vi "Open_File_for_write.vi"(8 "advisory dialog? (display:T)":bool=TRUE, 9 "append to file? (new file:F)":bool, 11 "file path":path) -> (0 "error out":errorcluster, 3 "refnum":refnum<file>)   [LabVIEW 2010]
doc: "Opens an existing file, creates a new file, or replaces an existing file, programmatically or interactively using dialog. You can optionally specify a dialog prompt, default file name, start path, or filter pattern, and you can specify open and deny modes when opening a file, plus group and permission when creating a new file. Use this VI with the intermediate Write File+ or Read File+ VIs described below.\n\nfile path is the path name of the file. If file path is empty (default value) or is Not A Path, the VI displays a File dialog box from which you can select a file. Error 43 occurs if the user cancels the dialog. \n\nfunction is the operation to perform:\n\n 0 (open) opens an existing file. Error 7 occurs if the file cannot be found.\n \n 1 (open or create) opens an existing file or creates a new file if one does not exist.\n\n 2 (create or replace) creates a new file or replaces a file if it exists and you give permission. Replacement is done by opening the file and setting EOF to 0. Error 43 occurs if the user elects to disallow the replacement using dialog. \n\n 3 (create) creates a new file. Error 8 occurs if the file already exists.\n\nadvisory dialog? Set TRUE (default) if you want a dialog if function=0 and the file does not exist, or if function=2 or 3 and the file exists.\n\nprompt is the message that appears below the list of files and directories in the file dialog.\n\ndefault name is the initial file name that appears in the selection box of the file dialog.\n\nstart path is the path name to the initially displayed directory in a file dialog. The default value is Not A Path, which is the path to the last directory shown in a file dialog.\n\npattern is the match pattern specification to display only certain types of files or directories. See the description of the File Dialog function for more information.\n\nerror in is a cluster of three elements (error?, code, and source) that describe the upstream error state, that is, the existance of any error preceeding the execution of the VI. The VI executes normally only if no incoming error exists; otherwise it merely passes the error in value to error out. error? is TRUE if an error occurred; the default value is FALSE. code is the error code; the default value is 0. source is in most cases the name of the VI or function that produced the error; the default value is an empty string.\n\nnew file path is the path of the file opened or created. You can use this output to determine the path of a file that you open or create using dialog. new file path returns Not A Path if the user selects Cancel from the dialog box.\n\nrefnum is the reference number of the open file. The value is Not A Refnum if the file cannot be opened.\n\nfile size is the size of the file in bytes; it is also the location of the end of file.\n\nerror out is a cluster of three elements (error?, code, and source) that describe the error state following the execution of the VI. If an incoming error does not exist, the VI executes normally and error out describes the VI's error state; if an incoming error exists, error out equals error in."
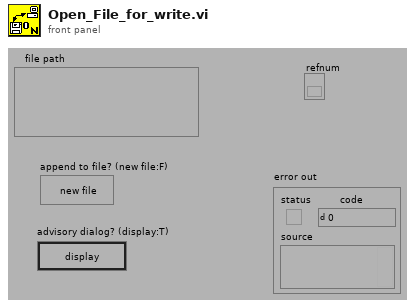
[diagram p1: front panel]
types:
  T1 = enum16{"deny read/write", "deny write-only", "deny none"}
  T2 = enum16{"read/write", "read-only", "write-only", "write-only (truncate)"}
  T3 = enum16{"open", "replace", "create", "open or create", "replace or create", "replace or create with confirmation"}
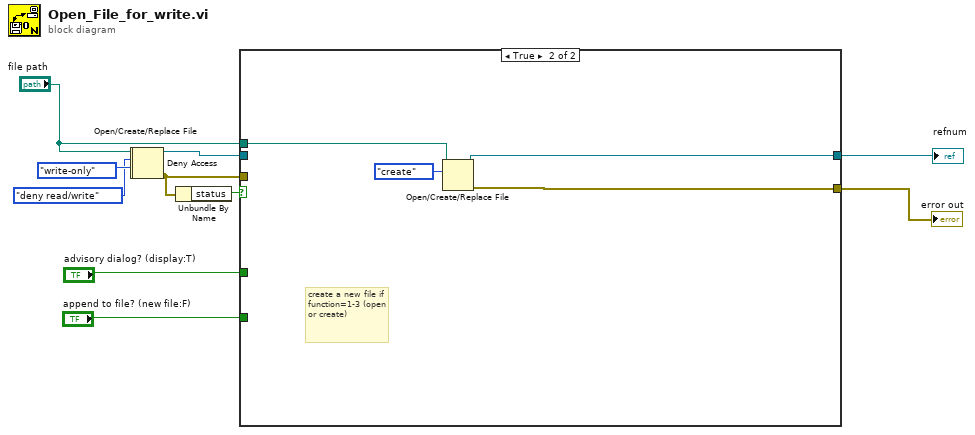
[diagram p0: block diagram]
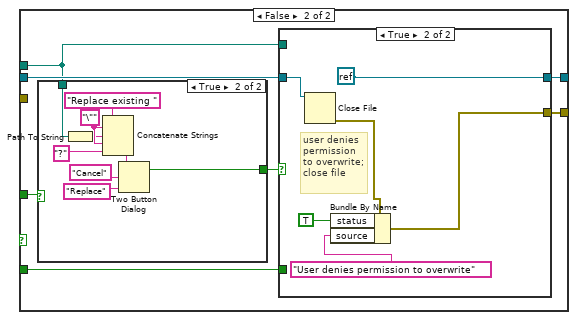
[diagram p3: hidden frame]
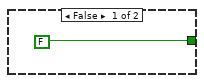
[diagram p4: hidden frame]
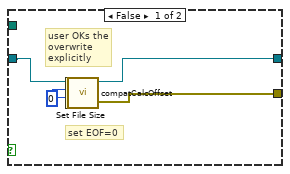
[diagram p5: hidden frame]
diagram:
  n1 = Open/Create/Replace File(file path (use dialog)="file path", access (0:read/write)=T2."write-only" ("open mode (0)")) -> (refnum out=w2:refnum<file>, error out=w3:errorcluster)  [unwired: 1 in, 4 out]
  n2 = Deny Access(4:w3, 6:T1."deny read/write" ("deny mode (2)"), 7:w2) -> (0:w7:errorcluster, 3:w11:refnum<file>)
  n3 = Unbundle By Name(w7) -> ("status"=w8:bool)
  n4 = case shown="True" w8 {
    tunnel: "file path" -> [w19 w53]
    tunnel: "append to file? (new file:F)" -> [w13 _]
    tunnel: [w18 w55] -> w10
    tunnel: w11 -> [w17 _]
    tunnel: "advisory dialog? (display:T)" -> [w16 _]
    tunnel: [w15 w54] -> w5
    tunnel: w7 -> [w14 _]
    frame False {
      # "file opened successfully"
      n5 = case shown="True" w13 {
        tunnel: w19 -> [_ w23]
        tunnel: [w21 w28] -> w18
        tunnel: w17 -> [w21 w27]
        tunnel: w16 -> [_ w25]
        tunnel: [w20 w24] -> w15
        tunnel: w14 -> [w20 _]
        tunnel: w13 -> [_ w22]
        frame True {
          # "file is now open; proceed if function=1 (open or create)"
        }
        frame False {
          n6 = case shown="True" w25 {
            tunnel: [FALSE w37] -> w26
            tunnel: w23 -> [_ w30]
            frame False {
            }
            frame True {
              w32 = "\""
              n7 = Path To String(path=w30) -> (string=w31:string)
              n8 = Concatenate Strings("Replace existing ", w32, w31, w32, "?") -> (w38:string)
              n9 = Two Button Dialog(message=w38, 1:"Replace", 2:"Cancel") -> (T button?=w37:bool)
            }
          }
          n10 = case shown="True" w26 {
            tunnel: [w43 refnum<k0> refnum] -> w28
            tunnel: w27 -> [w44 w50]
            tunnel: [w42 w46] -> w24
            tunnel: w23 -> [_ _]
            tunnel: w22 -> [_ _]
            frame False {
              w45 = 0
              # "user OKs the overwrite explicitly"
              # "set EOF=0"
              n11 = call <vilib>:"compatCalcOffset.vi"("pos offset (0)"=w45, "pos mode (0:1)"=w45, "refnum"=w44) -> ("error out"=w41:errorcluster, "offset"=w40:i32, "dup refnum"=w39:refnum<file>)  [unwired: 1 in, 5 out]
              n12 = Set File Size(4:w41, 6:w40, 7:w39) -> (0:w42:errorcluster, 3:w43:refnum<file>)
            }
            frame True {
              # "user denies permission to overwrite; close file"
              n13 = Close File(refnum=w50) -> (error out=w49:errorcluster)  [unwired: 1 in, 1 out]
              n14 = Bundle By Name(cluster=w49, "status"=TRUE, "source"="User denies permission to overwrite") -> (w46:errorcluster)
            }
          }
        }
      }
    }
    frame True {
      # "create a new file if function=1-3 (open or create)"
      n15 = Open/Create/Replace File(file path (use dialog)=w53, operation (0:open)=T3."create") -> (refnum out=w55:refnum<file>, error out=w54:errorcluster)  [unwired: 1 in, 4 out]
    }
  }
  "refnum" <- w10
  "error out" <- w5
